vi "LV SciSDK FRAME START.vi"(0 "Frame Name":string, 1 "Acq Mode":string(combo)="blocking", 2 "Timeout":i32=100, 3 "Thread":string(combo)="false", 4 "Board Handle In":T1, 5 "error in (no error)":errorcluster, 6 "High Performance":string(combo)="false", 7 "Trigger Mask":u32, 8 "Threaded Buffer Size":u32=100000, 9 "Wait Coincidence":u32, 10 "Trigger Mode":string(combo)="or", 11 "Sync Mode":string(combo)="master") -> (17 "Frame Handle Out":T2, 18 "Board Handle Out":T1, 19 "error out":errorcluster)   [LabVIEW 2021, in "SciSDK_Labview.lvlib"]
uses:
  SciSDK_Labview.lvlib
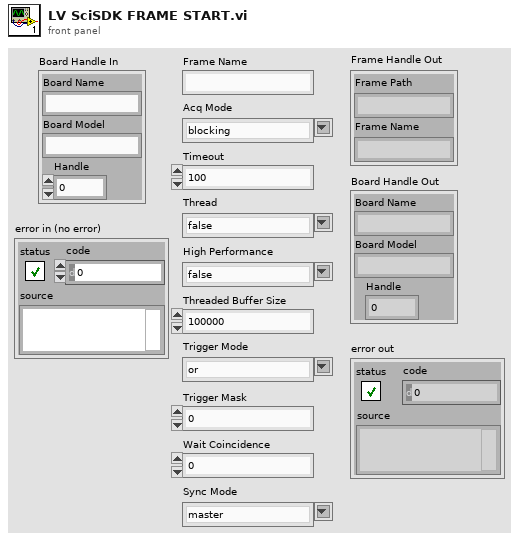
[diagram p1: front panel]
types:
  T1 = cluster{"Board Name":string, "Board Model":string, "Handle":u64}
  T2 = cluster{"Frame Path":string, "Frame Name":string}
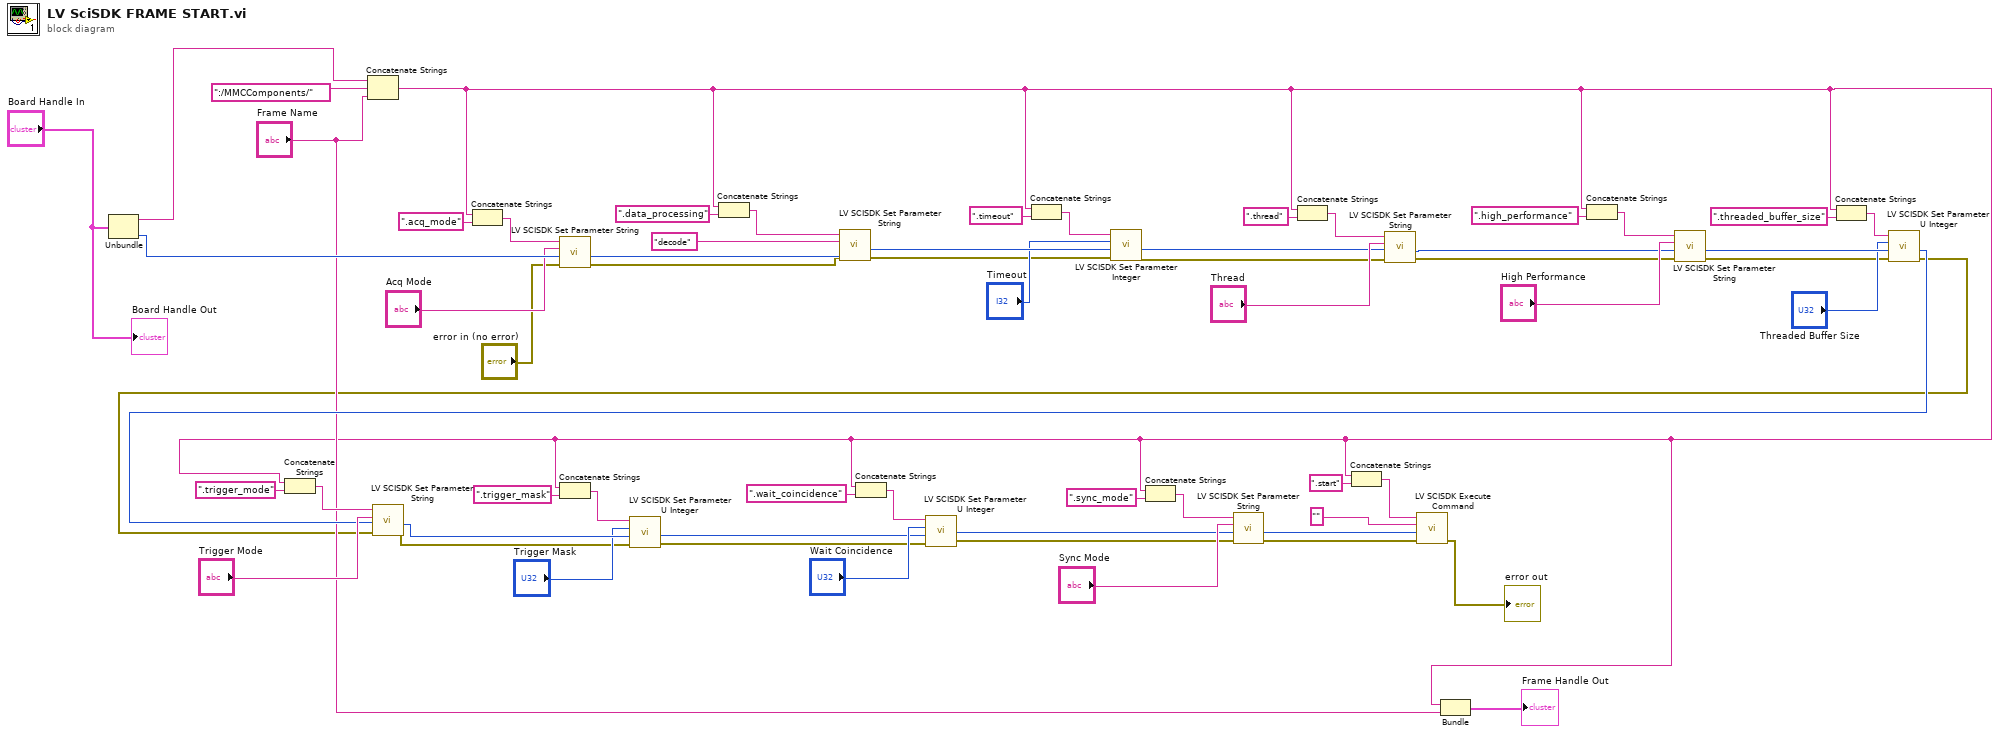
[diagram p0: block diagram]
diagram:
  n1 = Unbundle("Board Handle In") -> ("Board Name"=w61:string, "Handle"=w58:u64)  [unwired: 1 out]
  n2 = Concatenate Strings(w61, ":/MMCComponents/" ("string"), "Frame Name") -> (w3:string)
  n3 = Concatenate Strings(w3, ".trigger_mode" ("string")) -> (w36:string)
  n4 = Concatenate Strings(w3, ".acq_mode" ("string")) -> (w60:string)
  n5 = call "LV SCISDK Set Parameter String.vi"("error in (no error)"="error in (no error)", "handle"=w58, "value"="Acq Mode", "Path"=w60) -> ("error out"=w10:errorcluster, "handle out"=w53:u64)  [unwired: 5 in, 1 out]
  n6 = Concatenate Strings(w3, ".trigger_mask" ("string")) -> (w31:string)
  n7 = Concatenate Strings(w3, ".data_processing" ("string")) -> (w55:string)
  n8 = call "LV SCISDK Set Parameter String.vi"("error in (no error)"=w10, "handle"=w53, "value"="decode", "Path"=w55) -> ("error out"=w11:errorcluster, "handle out"=w52:u64)  [unwired: 5 in, 1 out]
  n9 = Concatenate Strings(w3, ".wait_coincidence" ("string")) -> (w27:string)
  n10 = Concatenate Strings(w3, ".timeout" ("string")) -> (w50:string)
  n11 = call "LV SCISDK Set Parameter Integer.vi"("error in (no error)"=w11, "handle"=w52, "value"="Timeout", "Path"=w50) -> ("error out"=w12:errorcluster, "handle out"=w45:u64)  [unwired: 5 in, 1 out]
  n12 = Concatenate Strings(w3, ".sync_mode" ("string")) -> (w24:string)
  n13 = Concatenate Strings(w3, ".thread" ("string")) -> (w48:string)
  n14 = Concatenate Strings(w3, ".start" ("string")) -> (w2:string)
  n15 = call "LV SCISDK Set Parameter String.vi"("error in (no error)"=w12, "handle"=w45, "value"="Thread", "Path"=w48) -> ("error out"=w13:errorcluster, "handle out"=w41:u64)  [unwired: 5 in, 1 out]
  n16 = Bundle(w3, "Frame Name"="Frame Name") -> (→"Frame Handle Out":cluster{string, "Frame Name":string})  [unwired: 1 in]
  n17 = Concatenate Strings(w3, ".high_performance" ("string")) -> (w44:string)
  n18 = call "LV SCISDK Set Parameter String.vi"("error in (no error)"=w13, "handle"=w41, "value"="High Performance", "Path"=w44) -> ("error out"=w14:errorcluster, "handle out"=w40:u64)  [unwired: 5 in, 1 out]
  n19 = Concatenate Strings(w3, ".threaded_buffer_size" ("string")) -> (w38:string)
  n20 = call "LV SCISDK Set Parameter U Integer.vi"("error in (no error)"=w14, "handle"=w40, "value"="Threaded Buffer Size", "Path"=w38) -> ("error out"=w15:errorcluster, "handle out"=w33:u64)  [unwired: 5 in, 1 out]
  n21 = call "LV SCISDK Set Parameter String.vi"("error in (no error)"=w15, "handle"=w33, "value"="Trigger Mode", "Path"=w36) -> ("error out"=w16:errorcluster, "handle out"=w30:u64)  [unwired: 5 in, 1 out]
  n22 = call "LV SCISDK Set Parameter U Integer.vi"("error in (no error)"=w16, "handle"=w30, "value"="Trigger Mask", "Path"=w31) -> ("error out"=w17:errorcluster, "handle out"=w25:u64)  [unwired: 5 in, 1 out]
  n23 = call "LV SCISDK Set Parameter U Integer.vi"("error in (no error)"=w17, "handle"=w25, "value"="Wait Coincidence", "Path"=w27) -> ("error out"=w18:errorcluster, "handle out"=w21:u64)  [unwired: 5 in, 1 out]
  n24 = call "LV SCISDK Set Parameter String.vi"("error in (no error)"=w18, "handle"=w21, "value"="Sync Mode", "Path"=w24) -> ("error out"=w7:errorcluster, "handle out"=w8:u64)  [unwired: 5 in, 1 out]
  n25 = call "LV SCISDK Execute Command.vi"("error in (no error)"=w7, "handle"=w8, "value"="", "Path"=w2) -> ("error out"=→"error out":errorcluster)  [unwired: 5 in, 2 out]
  "Board Handle Out" <- "Board Handle In"
